vi "createAckCMDEvent.vi"(8 "error in (no error)":errorcluster, 11 "PubSubDataEvent in":refnum<class "PubSubDataEvent.lvclass">) -> (0 "error out":errorcluster, 3 "PubSubDataEvent out":refnum<class "PubSubDataEvent.lvclass">)   [LabVIEW 2016, in "PubSubDataEvent.lvclass"]
uses:
  PubSubDataEvent.lvclass
  Typedefs/CommandValue.ctl
  PubSubDataEvent.lvclass/PubSubDataEvent.ctl
  Typedefs/EXATypedefs.lvlib
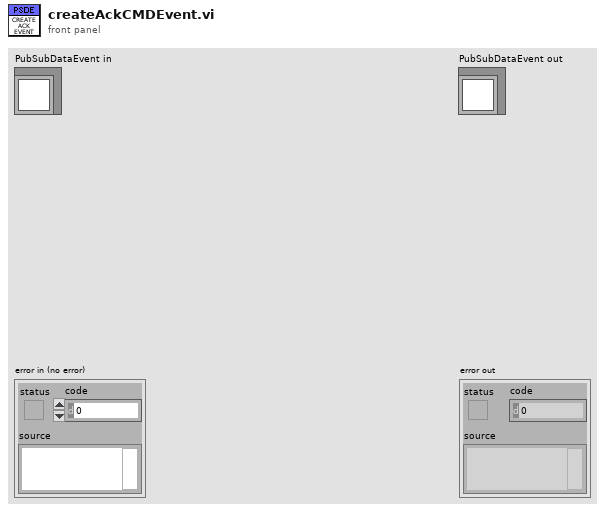
[diagram p1: front panel]
types:
  T1 = typedef "EXATypedefs.lvlib/CommandValue.ctl" = enum16{"ClearError", "Disable", "Enable", "Exit", "GoToStandby", "OnHeartbeat", "OnIncomingMessagingError", "OnInterrupt", "Start"}
  T2 = cluster{"error":i32, "result":string, "ack":i32, "cmdSeqNum":i32, "CommandValue":T1}
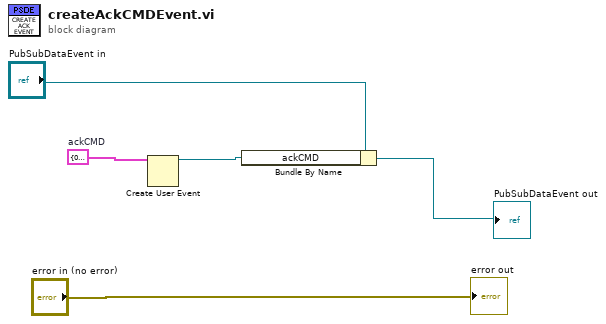
[diagram p0: block diagram]
diagram:
  w5 = T2 {"error"=0, "result"="", "ack"=0, "cmdSeqNum"=0, "CommandValue"=enum."ClearError"}  # ackCMD
  n1 = Create User Event(user event datatype=w5) -> (user event=w4:refnum<user-event>)  [unwired: 1 in, 1 out]
  n2 = Bundle By Name(cluster="PubSubDataEvent in", "ackCMD"=w4) -> (→"PubSubDataEvent out":refnum<class "PubSubDataEvent.lvclass">)
  "error out" <- "error in (no error)"
